vi "Init Drivetrain.vi"() -> (2 "Right Motors":T1={"DeviceStatus"={"status"=FALSE, "code"=0, "source"=""}, "Type"=enum."PWM", "PWM"={"PWM Channel"=enum."Invalid", "DeadBand"={"Name"="", "maxPositivePwm"=0, "minPositivePwm"=0, "centerPwm"=0, "maxNegativePwm"=0, "minNegativePwm"=0, "angularRange"=0}}, "CAN"={"Device Number"=0, "SetOutput VI Ref"=variant(refnum<vi> refnum), "GetOutput VI Ref"=variant(refnum<vi> refnum), "Enable VI Ref"=variant(refnum<vi> refnum), "Disable VI Ref"=variant(refnum<vi> refnum), "Data"=variant}, "Invert"=FALSE, "DIO PWM"={"PWM \"Enable\" Channel"=enum."Invalid", "DIOChannel"=enum."Invalid", "PWM Rate"=0.0}}, 3 "Left Motors":T1={"DeviceStatus"={"status"=FALSE, "code"=0, "source"=""}, "Type"=enum."PWM", "PWM"={"PWM Channel"=enum."Invalid", "DeadBand"={"Name"="", "maxPositivePwm"=0, "minPositivePwm"=0, "centerPwm"=0, "maxNegativePwm"=0, "minNegativePwm"=0, "angularRange"=0}}, "CAN"={"Device Number"=0, "SetOutput VI Ref"=variant(refnum<vi> refnum), "GetOutput VI Ref"=variant(refnum<vi> refnum), "Enable VI Ref"=variant(refnum<vi> refnum), "Disable VI Ref"=variant(refnum<vi> refnum), "Data"=variant}, "Invert"=FALSE, "DIO PWM"={"PWM \"Enable\" Channel"=enum."Invalid", "DIOChannel"=enum."Invalid", "PWM Rate"=0.0}})   [LabVIEW 2018]
uses:
  <vilib>/Rock Robotics/WPI/MotorControl/WPI_MotorControlDeviceRef.ctl
  <vilib>/Rock Robotics/WPI/MotorControl/WPI_MotorControlType.ctl
  <vilib>/Rock Robotics/SystemInterfaces/DIO/FPGA_DIOPWMChannel.ctl
  <vilib>/Rock Robotics/WPI/PWM/WPI_PWMDeadband.ctl
  <vilib>/Rock Robotics/SystemInterfaces/DIO/FPGA_DIOChannel.ctl
  <vilib>/Rock Robotics/WPI/ThirdParty/REV Robotics/SPARK MAX/Typedef/Spark MAX Motor Type.ctl
  <vilib>/Rock Robotics/WPI/ThirdParty/REV Robotics/SPARK MAX/Typedef/Spark MAX Idle Mode.ctl
panel:
  in  "Right Inverted":bool=TRUE
  in  "Left Inverted":bool
  in  "Right Master ID":u8=2
  in  "Right Talon ID":i32=2
  in  "Right Slave 2 ID":u8=6
  in  "Right Slave 1 ID":u8=4
  in  "Left Talon ID":i32=1
  in  "Left Slave 2 ID":u8=5
  in  "Left Slave 1 ID":u8=3
  in  "Left Master ID":u8=1
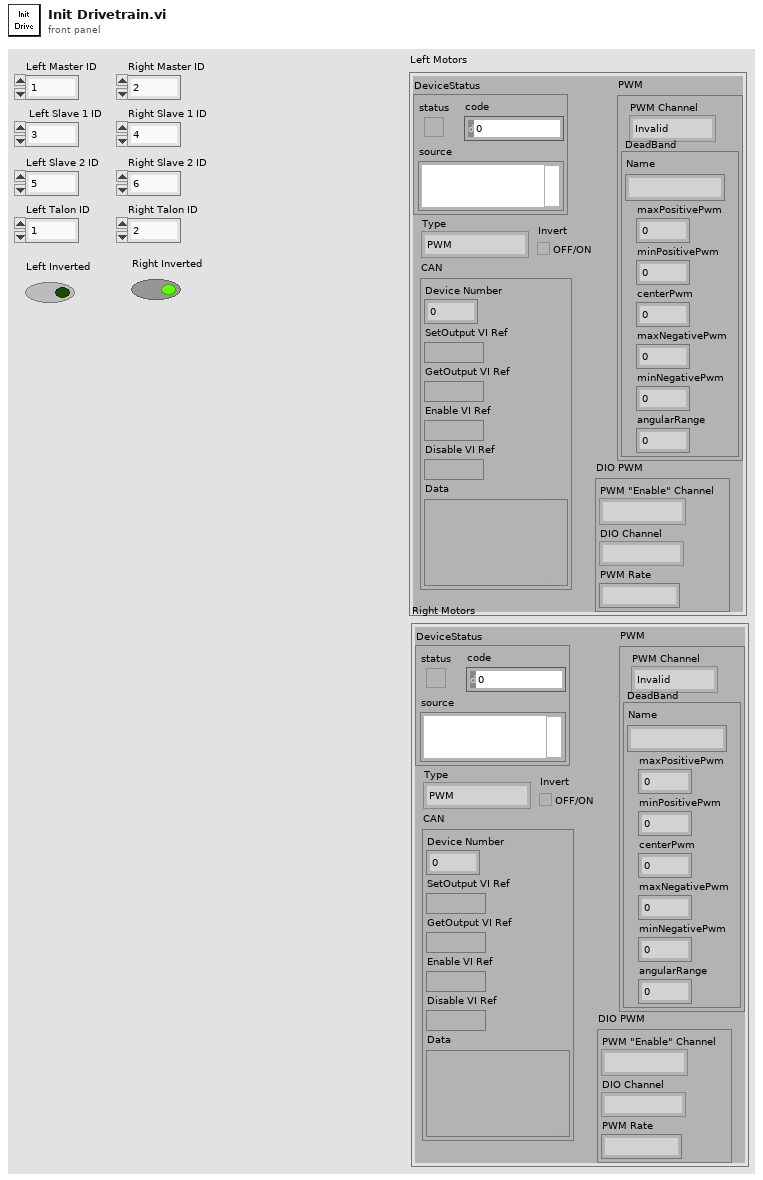
[diagram p1: front panel]
types:
  T1 = typedef "WPI_MotorControlDeviceRef.ctl" = cluster{"DeviceStatus":errorcluster, "Type":T2, "PWM":cluster{"PWM Channel":T3, "DeadBand":T4}, "CAN":cluster{"Device Number":u8, "SetOutput VI Ref":variant, "GetOutput VI Ref":variant, "Enable VI Ref":variant, "Disable VI Ref":variant, "Data":variant}, "Invert":bool, "DIO PWM":cluster{"PWM \"Enable\" Channel":T3, "DIOChannel":T5, "PWM Rate":dbl}}
  T2 = typedef "WPI_MotorControlType.ctl" = enum16{"PWM", "CAN", "DIO PWM"}
  T3 = typedef "FPGA_DIOPWMChannel.ctl" = enum8{"PWM 0", "PWM 1", "PWM 2", "PWM 3", "PWM 4", "PWM 5", "PWM 6", "PWM 7", "PWM 8", "PWM 9", "PWM MXP 0", "PWM MXP 1", "PWM MXP 2", "PWM MXP 3", "PWM MXP 4", "PWM MXP 5", "PWM MXP 6", "PWM MXP 7", "PWM MXP 8", "PWM MXP 9", "Invalid"}
  T4 = typedef "WPI_PWMDeadband.ctl" = cluster{"Name":string, "maxPositivePwm":i32, "minPositivePwm":i32, "centerPwm":i32, "maxNegativePwm":i32, "minNegativePwm":i32, "angularRange":u16}
  T5 = typedef "FPGA_DIOChannel.ctl" = enum8{"DIO 0", "DIO 1", "DIO 2", "DIO 3", "DIO 4", "DIO 5", "DIO 6", "DIO 7", "DIO 8", "DIO 9", "DIO MXP 0", "DIO MXP 1", "DIO MXP 2", "DIO MXP 3", "DIO MXP 4", "DIO MXP 5", "DIO MXP 6", "DIO MXP 7", "DIO MXP 8", "DIO MXP 9", "DIO MXP 10", "DIO MXP 11", "DIO MXP 12", "DIO MXP 13", "DIO MXP 14", "DIO MXP 15", "SPI Port CS1", "SPI Port CS2", "SPI Port CS3", "SPI Port MISO", "SPI Port MOSI", "Invalid"}
  T6 = typedef "Spark MAX Idle Mode.ctl" = enum16{"Coast", "Brake"}
  T7 = typedef "Spark MAX Motor Type.ctl" = enum16{"Brushed", "Brushless"}
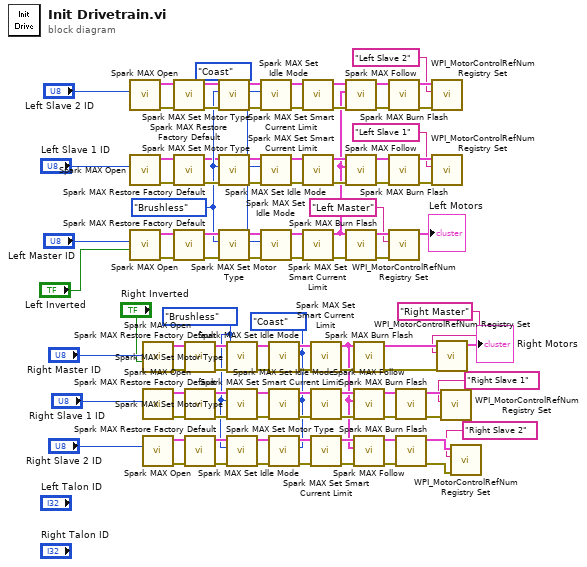
[diagram p0: block diagram]
diagram:
  w1 = Spark_MAX_Idle_Mode."Coast" ("Idle Mode")
  w2 = Spark_MAX_Idle_Mode."Coast" ("Idle Mode")
  w3 = Spark_MAX_Motor_Type."Brushless" ("Enum")
  w42 = Spark_MAX_Motor_Type."Brushless" ("Enum")
  n1 = call <vilib>:"Spark MAX Open.vi"("Device Number"="Left Slave 2 ID") -> ("error out"=w85:errorcluster, "MotorControlDeviceRef"=w35:T1)  [unwired: 9 in]
  n2 = call <vilib>:"Spark MAX Open.vi"("Device Number"="Left Slave 1 ID") -> ("error out"=w89:errorcluster, "MotorControlDeviceRef"=w36:T1)  [unwired: 9 in]
  n3 = call <vilib>:"Spark MAX Open.vi"("Invert"="Left Inverted", "Device Number"="Left Master ID") -> ("error out"=w93:errorcluster, "MotorControlDeviceRef"=w94:T1)  [unwired: 8 in]
  n4 = call <vilib>:"Spark MAX Open.vi"("Invert"="Right Inverted", "Device Number"="Right Master ID") -> ("error out"=w64:errorcluster, "MotorControlDeviceRef"=w65:T1)  [unwired: 8 in]
  n5 = call <vilib>:"Spark MAX Open.vi"("Device Number"="Right Slave 1 ID") -> ("error out"=w60:errorcluster, "MotorControlDeviceRef"=w33:T1)  [unwired: 9 in]
  n6 = call <vilib>:"Spark MAX Open.vi"("Device Number"="Right Slave 2 ID") -> ("error out"=w56:errorcluster, "MotorControlDeviceRef"=w26:T1)  [unwired: 9 in]
  n7 = call <vilib>:"Spark MAX Restore Factory Default.vi"("error in"=w85, "MotorControlDeviceRef"=w35) -> ("error out"=w86:errorcluster, "MotorControlDeviceRef"=w34:T1)  [unwired: 8 in]
  n8 = call <vilib>:"Spark MAX Restore Factory Default.vi"("error in"=w89, "MotorControlDeviceRef"=w36) -> ("error out"=w90:errorcluster, "MotorControlDeviceRef"=w37:T1)  [unwired: 8 in]
  n9 = call <vilib>:"Spark MAX Restore Factory Default.vi"("error in"=w93, "MotorControlDeviceRef"=w94) -> ("error out"=w95:errorcluster, "MotorControlDeviceRef"=w100:T1)  [unwired: 8 in]
  n10 = call <vilib>:"Spark MAX Restore Factory Default.vi"("error in"=w64, "MotorControlDeviceRef"=w65) -> ("error out"=w66:errorcluster, "MotorControlDeviceRef"=w71:T1)  [unwired: 8 in]
  n11 = call <vilib>:"Spark MAX Restore Factory Default.vi"("error in"=w60, "MotorControlDeviceRef"=w33) -> ("error out"=w61:errorcluster, "MotorControlDeviceRef"=w32:T1)  [unwired: 8 in]
  n12 = call <vilib>:"Spark MAX Restore Factory Default.vi"("error in"=w56, "MotorControlDeviceRef"=w26) -> ("error out"=w57:errorcluster, "MotorControlDeviceRef"=w27:T1)  [unwired: 8 in]
  n13 = call <vilib>:"Spark MAX Set Motor Type.vi"("error in (no error)"=w86, "Enum"=w42, "MotorControlDevRef"=w34) -> ("error out"=w87:errorcluster, "MotorControlDeviceRef"=w41:T1)  [unwired: 7 in]
  n14 = call <vilib>:"Spark MAX Set Motor Type.vi"("error in (no error)"=w90, "Enum"=w42, "MotorControlDevRef"=w37) -> ("error out"=w91:errorcluster, "MotorControlDeviceRef"=w38:T1)  [unwired: 7 in]
  n15 = call <vilib>:"Spark MAX Set Motor Type.vi"("error in (no error)"=w95, "Enum"=w42, "MotorControlDevRef"=w100) -> ("error out"=w96:errorcluster, "MotorControlDeviceRef"=w99:T1)  [unwired: 7 in]
  n16 = call <vilib>:"Spark MAX Set Motor Type.vi"("error in (no error)"=w66, "Enum"=w3, "MotorControlDevRef"=w71) -> ("error out"=w67:errorcluster, "MotorControlDeviceRef"=w70:T1)  [unwired: 7 in]
  n17 = call <vilib>:"Spark MAX Set Motor Type.vi"("error in (no error)"=w61, "Enum"=w3, "MotorControlDevRef"=w32) -> ("error out"=w62:errorcluster, "MotorControlDeviceRef"=w31:T1)  [unwired: 7 in]
  n18 = call <vilib>:"Spark MAX Set Motor Type.vi"("error in (no error)"=w57, "Enum"=w3, "MotorControlDevRef"=w27) -> ("error out"=w58:errorcluster, "MotorControlDeviceRef"=w28:T1)  [unwired: 7 in]
  n19 = call <vilib>:"Spark MAX Set Idle Mode.vi"("error in (no error)"=w87, "Idle Mode"=w1, "MotorControlDeviceRef in"=w41) -> ("error out"=w88:errorcluster, "MotorControlDeviceRef out"=w40:T1)  [unwired: 7 in]
  n20 = call <vilib>:"Spark MAX Set Idle Mode.vi"("error in (no error)"=w91, "Idle Mode"=w1, "MotorControlDeviceRef in"=w38) -> ("error out"=w92:errorcluster, "MotorControlDeviceRef out"=w39:T1)  [unwired: 7 in]
  n21 = call <vilib>:"Spark MAX Set Idle Mode.vi"("error in (no error)"=w96, "Idle Mode"=w1, "MotorControlDeviceRef in"=w99) -> ("error out"=w97:errorcluster, "MotorControlDeviceRef out"=w98:T1)  [unwired: 7 in]
  n22 = call <vilib>:"Spark MAX Set Idle Mode.vi"("error in (no error)"=w67, "Idle Mode"=w2, "MotorControlDeviceRef in"=w70) -> ("error out"=w68:errorcluster, "MotorControlDeviceRef out"=w69:T1)  [unwired: 7 in]
  n23 = call <vilib>:"Spark MAX Set Idle Mode.vi"("error in (no error)"=w62, "Idle Mode"=w2, "MotorControlDeviceRef in"=w31) -> ("error out"=w63:errorcluster, "MotorControlDeviceRef out"=w30:T1)  [unwired: 7 in]
  n24 = call <vilib>:"Spark MAX Set Idle Mode.vi"("error in (no error)"=w58, "Idle Mode"=w2, "MotorControlDeviceRef in"=w28) -> ("error out"=w59:errorcluster, "MotorControlDeviceRef out"=w29:T1)  [unwired: 7 in]
  n25 = call <vilib>:"Spark MAX Set Smart Current Limit.vi"("error in (no error)"=w88, "MotorControlDeviceRef in"=w40) -> ("error out"=w77:errorcluster, "MotorControlDeviceRef out"=w80:T1)  [unwired: 8 in]
  n26 = call <vilib>:"Spark MAX Set Smart Current Limit.vi"("error in (no error)"=w92, "MotorControlDeviceRef in"=w39) -> ("error out"=w75:errorcluster, "MotorControlDeviceRef out"=w81:T1)  [unwired: 8 in]
  n27 = call <vilib>:"Spark MAX Set Smart Current Limit.vi"("error in (no error)"=w97, "MotorControlDeviceRef in"=w98) -> ("error out"=w74:errorcluster, "MotorControlDeviceRef out"=w73:T1)  [unwired: 8 in]
  n28 = call <vilib>:"Spark MAX Set Smart Current Limit.vi"("error in (no error)"=w68, "MotorControlDeviceRef in"=w69) -> ("error out"=w48:errorcluster, "MotorControlDeviceRef out"=w47:T1)  [unwired: 8 in]
  n29 = call <vilib>:"Spark MAX Set Smart Current Limit.vi"("error in (no error)"=w63, "MotorControlDeviceRef in"=w30) -> ("error out"=w49:errorcluster, "MotorControlDeviceRef out"=w55:T1)  [unwired: 8 in]
  n30 = call <vilib>:"Spark MAX Set Smart Current Limit.vi"("error in (no error)"=w59, "MotorControlDeviceRef in"=w29) -> ("error out"=w51:errorcluster, "MotorControlDeviceRef out"=w54:T1)  [unwired: 8 in]
  n31 = call <vilib>:"Spark MAX Follow.vi"("error in (no error)"=w77, "Master Controller"=w73, "MotorControlDeviceRef"=w80) -> ("error out"=w78:errorcluster, "MotorControlDeviceRef"=w79:T1)  [unwired: 7 in]
  n32 = call <vilib>:"Spark MAX Follow.vi"("error in (no error)"=w75, "Master Controller"=w73, "MotorControlDeviceRef"=w81) -> ("error out"=w76:errorcluster, "MotorControlDeviceRef"=w72:T1)  [unwired: 7 in]
  n33 = call <vilib>:"Spark MAX Burn Flash.vi"("error in"=w74, "MotorControlDeviceRef"=w73) -> ("error out"=w16:errorcluster, "MotorControlDeviceRef"=w17:T1)  [unwired: 8 in]
  n34 = call <vilib>:"Spark MAX Burn Flash.vi"("error in"=w48, "MotorControlDeviceRef"=w47) -> ("error out"=w23:errorcluster, "MotorControlDeviceRef"=w25:T1)  [unwired: 8 in]
  n35 = call <vilib>:"Spark MAX Follow.vi"("error in (no error)"=w49, "Master Controller"=w47, "MotorControlDeviceRef"=w55) -> ("error out"=w50:errorcluster, "MotorControlDeviceRef"=w46:T1)  [unwired: 7 in]
  n36 = call <vilib>:"Spark MAX Follow.vi"("error in (no error)"=w51, "Master Controller"=w47, "MotorControlDeviceRef"=w54) -> ("error out"=w52:errorcluster, "MotorControlDeviceRef"=w53:T1)  [unwired: 7 in]
  n37 = call <vilib>:"Spark MAX Burn Flash.vi"("error in"=w78, "MotorControlDeviceRef"=w79) -> ("error out"=w10:errorcluster, "MotorControlDeviceRef"=w11:T1)  [unwired: 8 in]
  n38 = call <vilib>:"Spark MAX Burn Flash.vi"("error in"=w76, "MotorControlDeviceRef"=w72) -> ("error out"=w13:errorcluster, "MotorControlDeviceRef"=w14:T1)  [unwired: 8 in]
  n39 = call <vilib>:"WPI_MotorControlRefNum Registry Set.vi"("error in (no error)"=w16, "refnum name"="Left Master", "MotorControlDevRef"=w17) -> ("MotorControlDevRef"=→"Left Motors":T1)  [unwired: 7 in, 1 out]
  n40 = call <vilib>:"Spark MAX Burn Flash.vi"("error in"=w50, "MotorControlDeviceRef"=w46) -> ("error out"=w21:errorcluster, "MotorControlDeviceRef"=w22:T1)  [unwired: 8 in]
  n41 = call <vilib>:"Spark MAX Burn Flash.vi"("error in"=w52, "MotorControlDeviceRef"=w53) -> ("error out"=w8:errorcluster, "MotorControlDeviceRef"=w19:T1)  [unwired: 8 in]
  n42 = call <vilib>:"WPI_MotorControlRefNum Registry Set.vi"("error in (no error)"=w10, "refnum name"="Left Slave 2", "MotorControlDevRef"=w11) -> ()  [unwired: 7 in, 2 out]
  n43 = call <vilib>:"WPI_MotorControlRefNum Registry Set.vi"("error in (no error)"=w13, "refnum name"="Left Slave 1", "MotorControlDevRef"=w14) -> ()  [unwired: 7 in, 2 out]
  n44 = call <vilib>:"WPI_MotorControlRefNum Registry Set.vi"("error in (no error)"=w23, "refnum name"="Right Master", "MotorControlDevRef"=w25) -> ("MotorControlDevRef"=→"Right Motors":T1)  [unwired: 7 in, 1 out]
  n45 = call <vilib>:"WPI_MotorControlRefNum Registry Set.vi"("error in (no error)"=w21, "refnum name"="Right Slave 1", "MotorControlDevRef"=w22) -> ()  [unwired: 7 in, 2 out]
  n46 = call <vilib>:"WPI_MotorControlRefNum Registry Set.vi"("error in (no error)"=w8, "refnum name"="Right Slave 2", "MotorControlDevRef"=w19) -> ()  [unwired: 7 in, 2 out]
